vi "SetWindowMouseRect.vi"(8 "No Error":errorcluster, 9 "Rect":T1, 10 "Destroy Previously Set Barrier":bool, 11 "Window [SDL_Window *]":T2 format="%.0x") -> (0 "Error Out":errorcluster)   [LabVIEW 2026, in "SDL3.lvlib" / "Video.lvlib"]
doc: "<B>Summary</B>\nConfines the cursor to the specified area of a window.\n\n<B>Remarks</B>\nNote that this does NOT grab the cursor, it only defines the area a cursor is restricted to when the window has mouse focus."
uses:
  Video.lvlib
  Rect/Rect--cluster.ctl
  <vilib>/Utility/error.llb/Error Cluster From Error Code.vi
  Error/Error.lvlib
  Lib/SDL3.dll
  Rect/Rect.lvlib
  SDL_Window--pointer.ctl
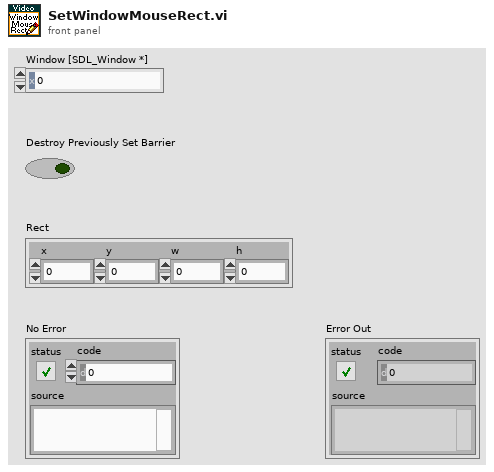
[diagram p1: front panel]
types:
  T1 = typedef "SDL3.lvlib/Rect.lvlib/Rect--cluster.ctl" = cluster{"x":i32, "y":i32, "w":i32, "h":i32}
  T2 = typedef "SDL3.lvlib/Video.lvlib/SDL_Window--pointer.ctl" = i64
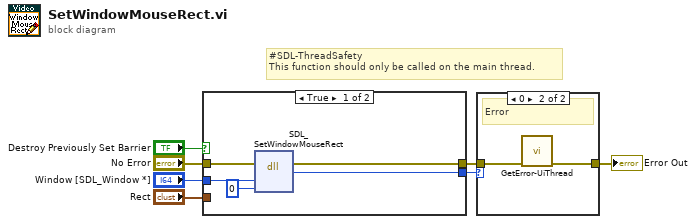
[diagram p0: block diagram]
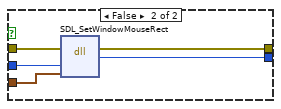
[diagram p2: hidden frame]
diagram:
  # "#SDL-ThreadSafety\nThis function should only be called on the main thread."
  n1 = case shown="True" "Destroy Previously Set Barrier" {
    tunnel: "No Error" -> [w12 w17]
    tunnel: "Window [SDL_Window *]" -> [w11 w16]
    tunnel: [w10 w15] -> w4
    tunnel: [w9 w14] -> w3
    tunnel: "Rect" -> [_ w13]
    frame True {
      n2 = dll-call lib="C:/Users/saukko/Dev/LV-SDL3/Sources/SDL3/Lib/SDL3.*" fn="SDL_SetWindowMouseRect"(error in=w12, "window"=w11, "rect"=i64 0) -> (error out=w10:errorcluster, "return type"=w9:i32)  [unwired: 4 in, 1 out]
    }
    frame False {
      n3 = dll-call lib="C:/Users/saukko/Dev/LV-SDL3/Sources/SDL3/Lib/SDL3.*" fn="SDL_SetWindowMouseRect"(error in=w17, "window"=w16, "rect"=w13) -> (error out=w15:errorcluster, "return type"=w14:i32)  [unwired: 4 in, 1 out]
    }
  }
  n4 = case shown="0" w3 {
    tunnel: w4 -> [w18 w20]
    tunnel: [w18 w19] -> w6
    frame Default {
      # "Ok"
    }
    frame 0 {
      # "Error"
      n5 = call "GetError-UiThread.vi"("No Error"=w20) -> ("error out"=w19:errorcluster)  [unwired: 10 in]
    }
  }
  "Error Out" <- w6
